vi "Data_Open.vi"(8 "Error In":errorcluster caption="错误输入", 11 "文件路径（使用对话框）":path) -> (0 "Error Out":errorcluster caption="错误输出", 3 "数据文件对象":refnum<file>)   [LabVIEW 2020]
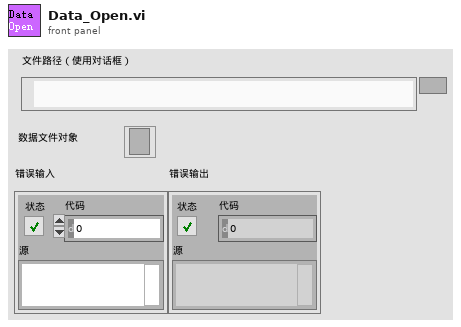
[diagram p1: front panel]
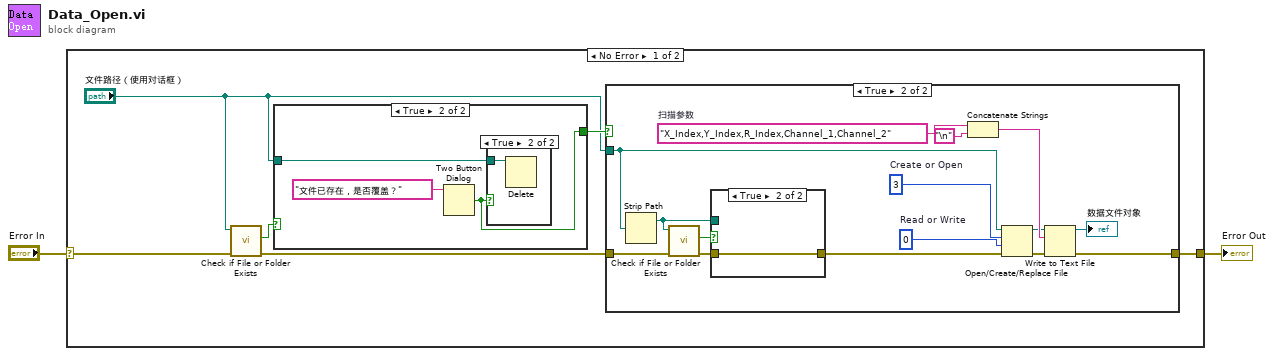
[diagram p0: block diagram]
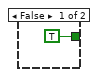
[diagram p2: hidden frame]
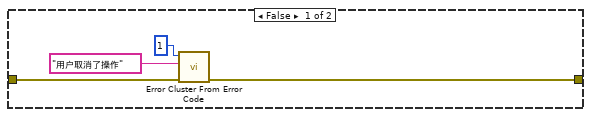
[diagram p4: hidden frame]
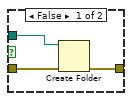
[diagram p5: hidden frame]
diagram:
  n1 = case shown="No Error" "Error In" {
    selector: "Error In" -> [w7 w37]
    tunnel: [w8 w37] -> w1
    frame No Error {
      n2 = call <vilib>:"Check if File or Folder Exists.vi"("error in (no error)"=w7, "path"="文件路径（使用对话框）") -> ("error out"=w6:errorcluster, "file or folder exists?"=w5:bool)  [unwired: 7 in, 1 out]
      n3 = case shown="True" w5 {
        tunnel: [TRUE w11] -> w4
        tunnel: "文件路径（使用对话框）" -> [_ w10]
        frame False {
        }
        frame True {
          n4 = Two Button Dialog(message="文件已存在，是否覆盖？") -> (T button?=w11:bool)  [unwired: 2 in]
          n5 = case shown="True" w11 {
            tunnel: w10 -> [_ w13]
            frame False {
            }
            frame True {
              n6 = Delete(path (use dialog)=w13) -> ()  [unwired: 4 in, 3 out]
            }
          }
        }
      }
      n7 = case shown="True" w4 {
        tunnel: [w17 w29] -> w8
        tunnel: "文件路径（使用对话框）" -> [_ w20]
        tunnel: w6 -> [w16 w19]
        frame False {
          n8 = call <vilib>:"Error Cluster From Error Code.vi"("error in (no error)"=w16, "error message (\"\")"="用户取消了操作", "error code (0)"=1) -> ("error out"=w17:errorcluster)  [unwired: 6 in]
        }
        frame True {
          w25 = "X_Index,Y_Index,R_Index,Channel_1,Channel_2"  # 扫描参数
          w31 = 0  # Read or Write
          w32 = 3  # Create or Open
          n9 = Strip Path(path=w20) -> (stripped path=w21:path)  [unwired: 1 out]
          n10 = call <vilib>:"Check if File or Folder Exists.vi"("error in (no error)"=w19, "path"=w21) -> ("error out"=w18:errorcluster, "file or folder exists?"=w22:bool)  [unwired: 7 in, 1 out]
          n11 = case shown="True" w22 {
            tunnel: w18 -> [w35 w36]
            tunnel: [w34 w36] -> w24
            tunnel: w21 -> [w33 _]
            frame False {
              n12 = Create Folder(path (use dialog)=w33, error in=w35) -> (error out=w34:errorcluster)  [unwired: 1 in, 2 out]
            }
            frame True {
            }
          }
          n13 = Concatenate Strings(w25, "\n") -> (w28:string)
          n14 = Open/Create/Replace File(file path (use dialog)=w20, error in=w24, operation (0:open)=w32, access (0:read/write)=w31) -> (refnum out=w26:refnum<file>, error out=w30:errorcluster)  [unwired: 2 in, 1 out]
          n15 = Write to Text File(file (use dialog)=w26, text=w28, error in=w30) -> (refnum out=→"数据文件对象":refnum<file>, error out=w29:errorcluster)  [unwired: 1 in, 1 out]
        }
      }
    }
    frame Error {
    }
  }
  "Error Out" <- w1
